vi "All_stats.vi"(3 "Timescales":dbl[](array[numeric]), 4 "Equi Spaced":dbl[][](array[numeric]) format="%.2f", 5 "LDA":dbl[][](array[numeric]) format="%.2f") -> (1 "Stats array":string[](array[string]))   [LabVIEW 2010]
uses:
  Globals/LDA_meas_global_1.vi
  Globals/Meas_global.vi
  Acquisition/PWA/PWAtasksGLOBAL.vi
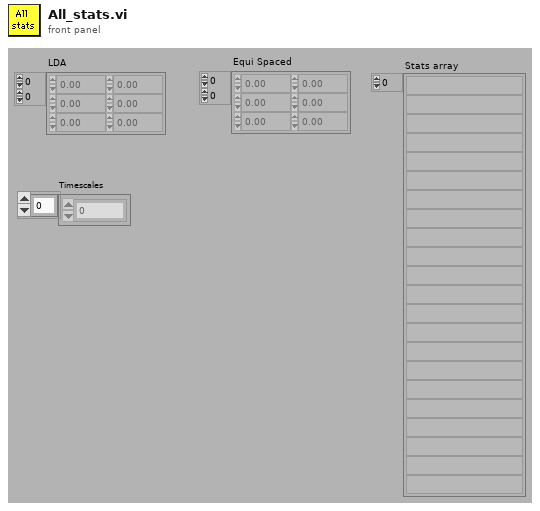
[diagram p1: front panel]
types:
  T1 = typedef "Analysis_type_cluster.ctl" = cluster{"Analysis type":T2, "Indicies":i32[], "Name":string, "Inst Array":T3, "Info index":i32}
  T2 = typedef "Analysis_type_Enum.ctl" = enum16{"Slow Response", "Fast Response", "Weighted Fast Response", "Fast FID", "Weighted Fast FID", "Cross Wire", "Weighted Cross Wire", "Weighted LDA"}
  T3 = typedef "Instrument_Array.ctl" = enum16{"PWA", "LDA", "Analogue"}
  T4 = typedef "Analysis_info_cluster.ctl" = cluster{"Colour":u32, "Inst type":T5, "Inst name":string, "Symbol":string, "Code name":string, "Extra Info":string, "Inst Array":T3, "Index":i32, "Voltage Index":i32, "Extra Titles":string[], "Extra Values":string[]}
  T5 = typedef "Inst_type.ctl" = enum16{"Propeller anemometer", "Raw voltage", "Pressure Transducer", "Pitot-static tube", "Preston tube", "Hot wire", "Cross wire 1", "Cross wire 2", "Generic Linear", "Generic Polynomial", "Generic BackPoly", "Fast FID", "Thermocouple", "Cold wire", "Pulsed Wire", "LDA Vel", "LDA Tran time", "LDA Arr time"}
  T6 = typedef "Velocity_cluster.ctl" = cluster{"Name":string, "U":dbl, "u^2":dbl, "u^3/(u^2)^(1.5)":dbl, "u^4/(u^2)^2 -3":dbl, "% u'/U":dbl, "Mean % Err":dbl, "u^4":dbl}
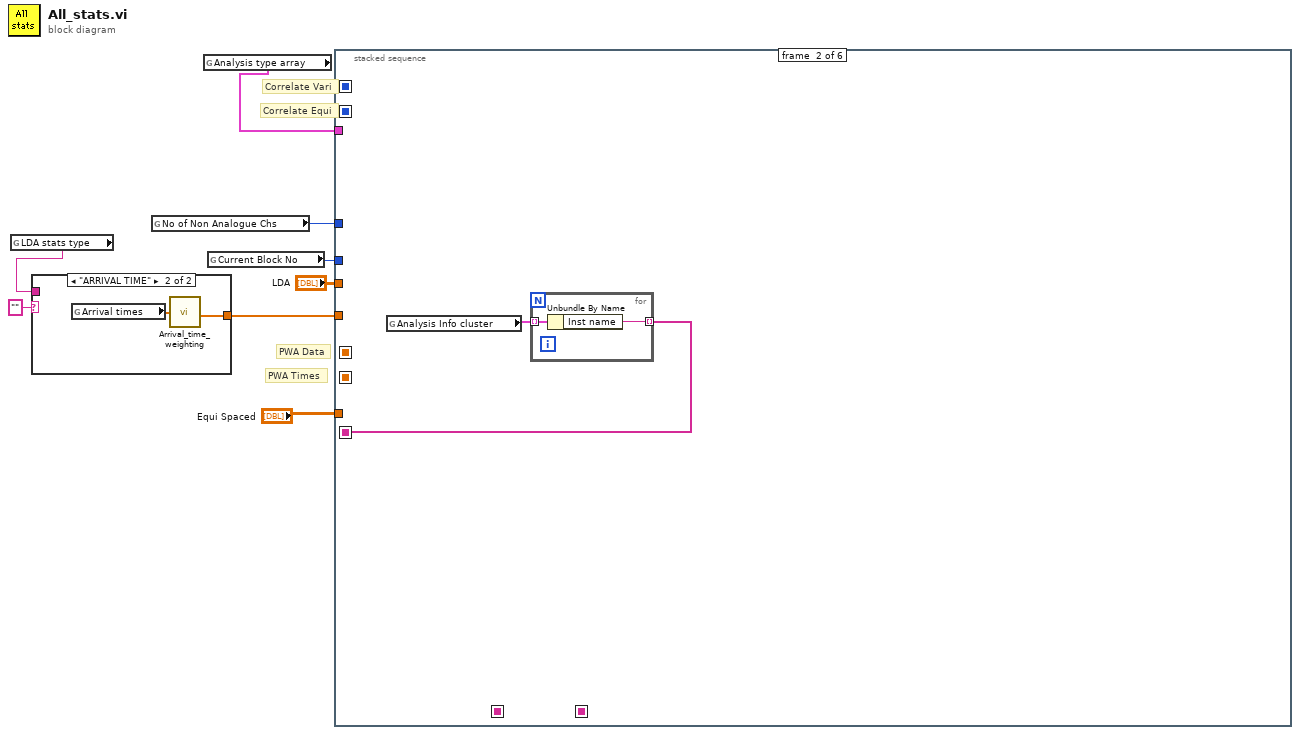
[diagram p0: block diagram]
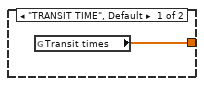
[diagram p2: hidden frame]
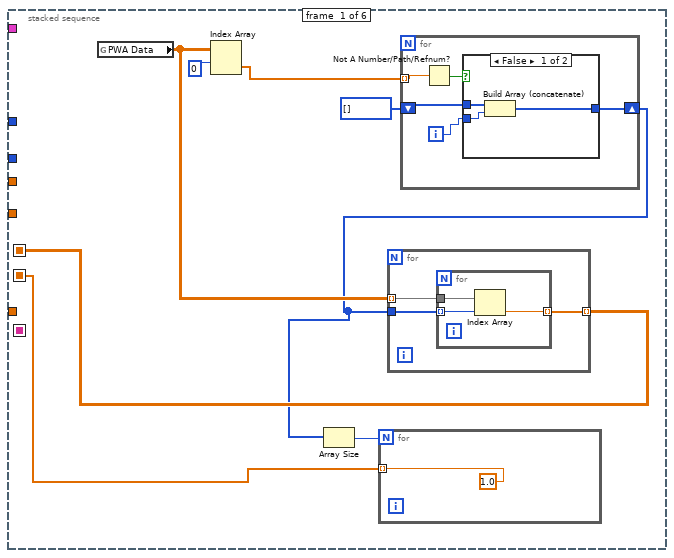
[diagram p3: hidden frame]
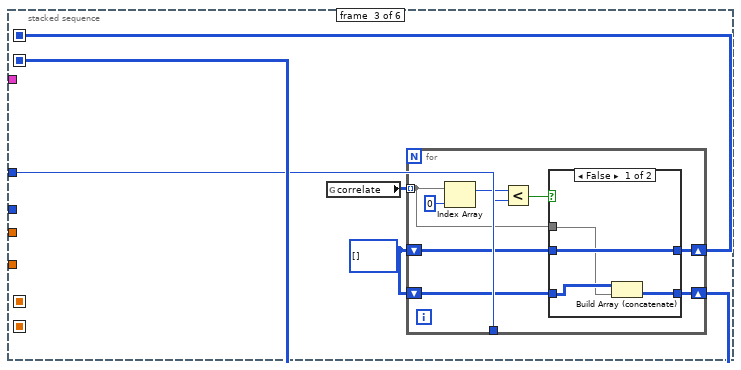
[diagram p5: hidden frame]
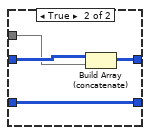
[diagram p6: hidden frame]
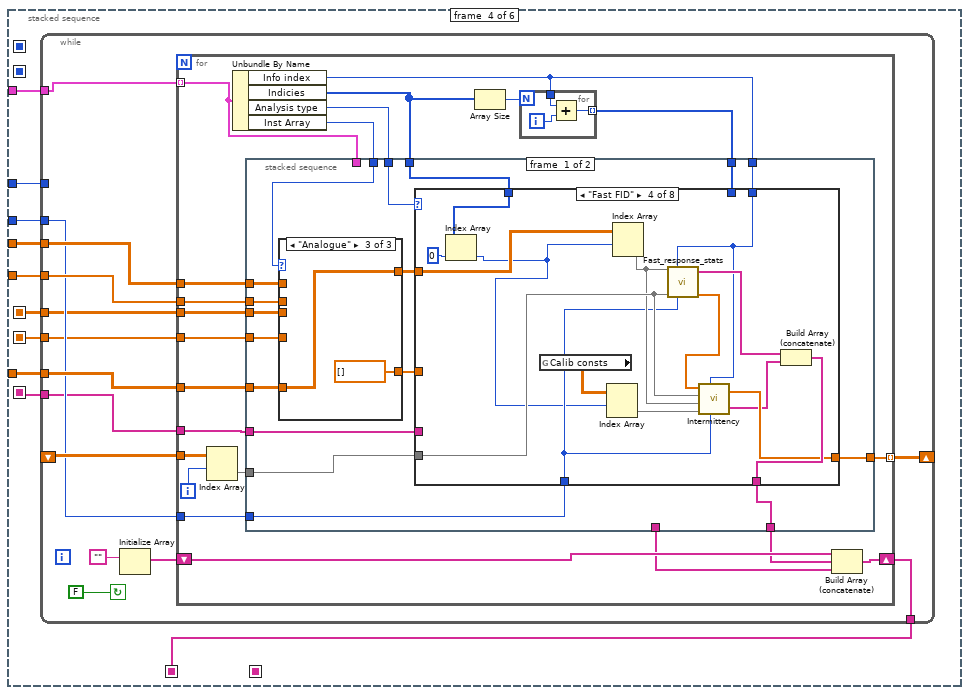
[diagram p7: hidden frame]
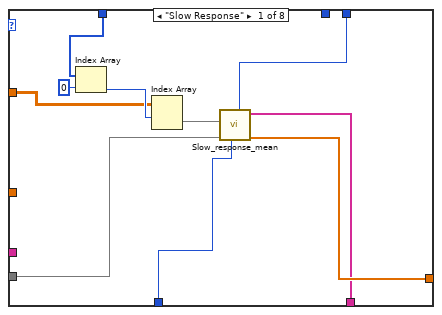
[diagram p10: hidden frame]
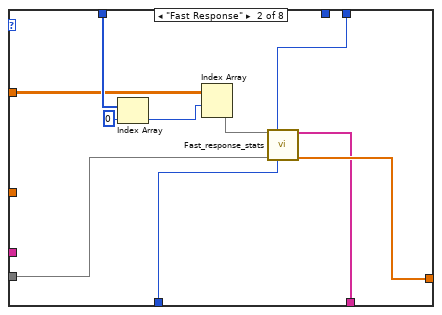
[diagram p11: hidden frame]
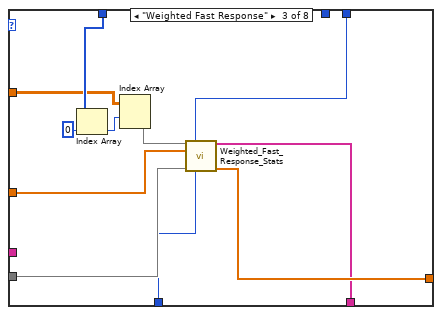
[diagram p12: hidden frame]
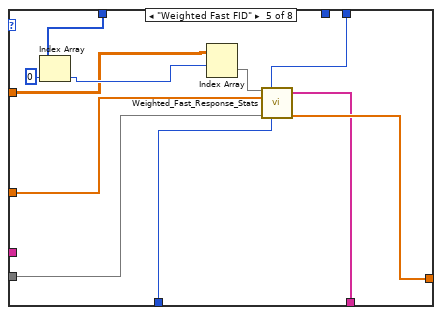
[diagram p13: hidden frame]
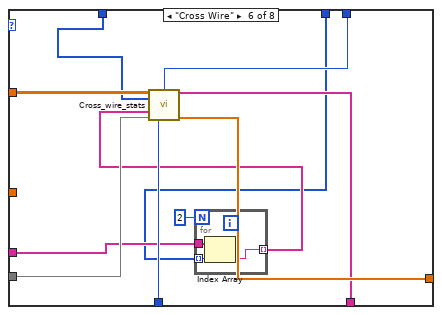
[diagram p14: hidden frame]
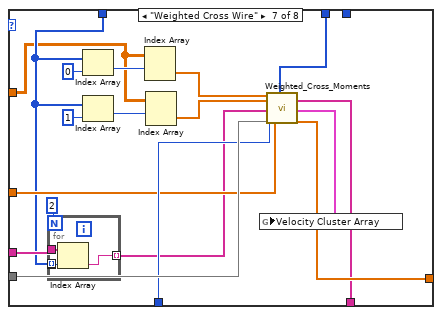
[diagram p15: hidden frame]
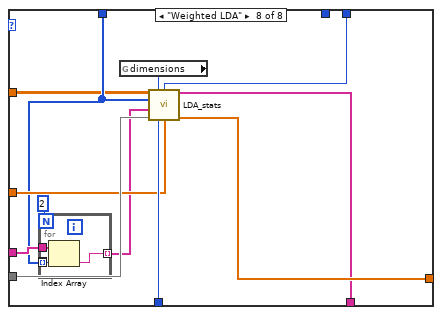
[diagram p16: hidden frame]
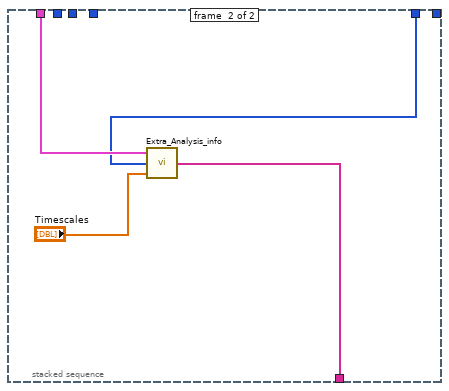
[diagram p17: hidden frame]
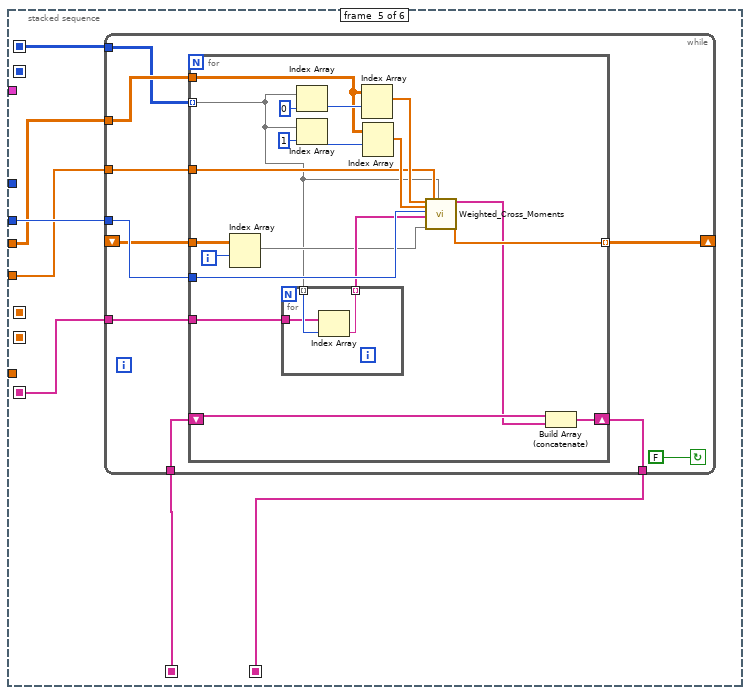
[diagram p18: hidden frame]
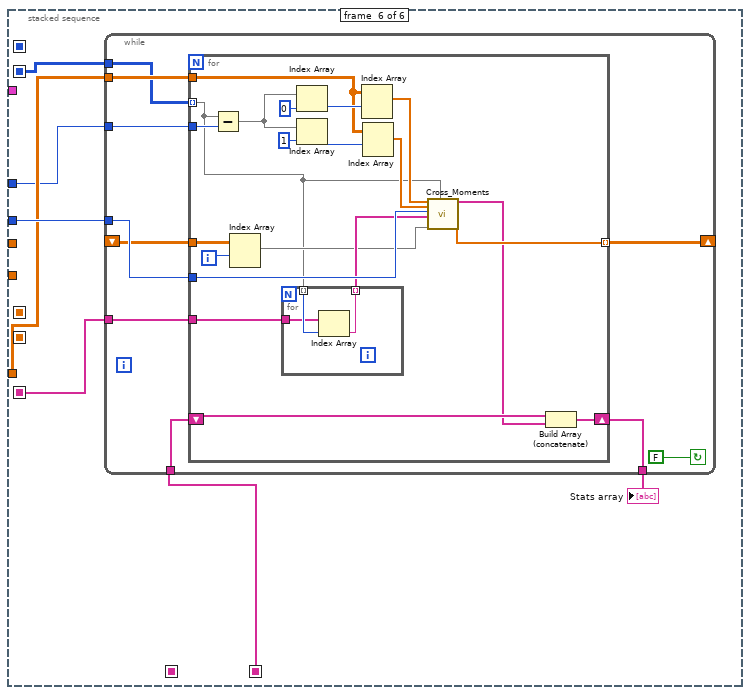
[diagram p19: hidden frame]
diagram:
  # "PWA Times"
  # "PWA Data"
  # "Correlate Equi"
  # "Correlate Vari"
  n1 = global read "LDA_meas_global_1.vi" "LDA stats type"() -> (w1:string)
  n2 = case shown="\"ARRIVAL TIME\"" "" {
    tunnel: [w9 w10] -> w4
    tunnel: w1 -> [_ _]
    frame "TRANSIT TIME", Default {
      n3 = global read "LDA_meas_global_1.vi" "Transit times"() -> (w9:dbl[])
    }
    frame "ARRIVAL TIME" {
      n4 = global read "LDA_meas_global_1.vi" "Arrival times"() -> (w11:dbl[])
      n5 = call "Arrival_time_weighting.vi"("Arrival times"=w11) -> ("Weighting"=w10:dbl[])
    }
  }
  n6 = global read "Meas_global.vi" "No of Non Analogue Chs"() -> (w5:i32)
  n7 = global read "Meas_global.vi" "Analysis type array"() -> (w3:T1[])
  n8 = global read "Meas_global.vi" "Current Block No"() -> (w8:i32)
  n9 = stacked-sequence {
    seq-local: [_ _ _ w69 _ _] -> [_ _ _ _ w249 _]
    seq-local: [_ w36 _ _ _ _] -> [_ _ _ w66 w246 w289]
    seq-local: [_ _ w42 _ _ _] -> [_ _ _ _ w248 _]
    seq-local: [_ _ w41 _ _ _] -> [_ _ _ _ _ w286]
    seq-local: [_ _ _ _ w247 _] -> [_ _ _ _ _ w288]
    seq-local: [w15 _ _ _ _ _] -> [_ _ _ w63 _ _]
    seq-local: [w12 _ _ _ _ _] -> [_ _ _ w62 _ _]
    tunnel: w8 -> [_ _ _ w71 w251 w290]
    tunnel: "LDA" -> [_ _ _ w70 w250 _]
    tunnel: "Equi Spaced" -> [_ _ _ w68 _ w285]
    tunnel: w4 -> [_ _ _ w67 w245 _]
    tunnel: w5 -> [_ _ w40 w64 _ w284]
    tunnel: w3 -> [_ _ _ w65 _ _]
    frame #0 {
      n10 = global read "PWAtasksGLOBAL.vi" "PWA Data"() -> (w16:dbl[][])
      n11 = Index Array(array=w16, index (row)=0) -> (element=w18:dbl[])  [unwired: 1 in]
      n12 = for {
        tunnel: w18 -> [w28] mode=indexing
        shift-right: [w30] -> w14
        shift-left: i32[] [] -> [w31]
        i -> [w27]
        n13 = Not A Number/Path/Refnum?(number/path/refnum=w28) -> (NaN/Path/Refnum?=w29:bool)
        n14 = case shown="False" w29 {
          tunnel: w31 -> [w34 w35]
          tunnel: [w33 w35] -> w30
          tunnel: w27 -> [w32 _]
          frame False {
            n15 = Build Array (concatenate)(w34, w32) -> (w33:i32[])
          }
          frame True {
          }
        }
      }
      n16 = Array Size(array=w14) -> (size(s)=w13:i32)
      n17 = for {
        N: w13 -> [_]
        tunnel: [1.0] -> w12 mode=indexing
      }
      n18 = for {
        tunnel: w14 -> [w23]
        tunnel: w16 -> [w22] mode=indexing
        tunnel: [w21] -> w15 mode=indexing
        n19 = for {
          tunnel: w23 -> [w26] mode=indexing
          tunnel: w22 -> [w25]
          tunnel: [w24] -> w21 mode=indexing
          n20 = Index Array(array=w25, index=w26) -> (element=w24:dbl)
        }
      }
    }
    frame #1 {
      n21 = global read "Meas_global.vi" "Analysis Info cluster"() -> (w37:T4[])
      n22 = for {
        tunnel: w37 -> [w39] mode=indexing
        tunnel: [w38] -> w36 mode=indexing
        n23 = Unbundle By Name(w39) -> ("Inst name"=w38:string)
      }
    }
    frame #2 {
      w43 = i32[][] []
      n24 = global read "Meas_global.vi" "correlate"() -> (w44:i32[][])
      n25 = for {
        tunnel: w44 -> [w49] mode=indexing
        tunnel: w40 -> [w45]
        shift-right: [w48] -> w42
        shift-left: w43 -> [w50]
        shift-right: [w46] -> w41
        shift-left: w43 -> [w47]
        n26 = Index Array(array=w49, index=0 ("Index")) -> (element=w52:i32)
        n27 = Less?(x=w52, y=w45) -> (x < y?=w51:bool)
        n28 = case shown="False" w51 {
          tunnel: w50 -> [w55 w61]
          tunnel: w49 -> [w54 w60]
          tunnel: [w55 w59] -> w48
          tunnel: w47 -> [w57 w58]
          tunnel: [w56 w58] -> w46
          frame False {
            n29 = Build Array (concatenate)(w57, w54) -> (w56:i32[][])
          }
          frame True {
            n30 = Build Array (concatenate)(w61, w60) -> (w59:i32[][])
          }
        }
      }
    }
    frame #3 {
      n31 = while {
        tunnel: w66 -> [w76]
        tunnel: w67 -> [w79]
        tunnel: w68 -> [w81]
        tunnel: [w82] -> w69
        shift-left: _ -> [w78]
        shift-right: [w85] -> _
        tunnel: w70 -> [w80]
        tunnel: w71 -> [w77]
        tunnel: w65 -> [w74]
        tunnel: w64 -> [_]
        tunnel: w63 -> [w73]
        tunnel: w62 -> [w72]
        stop <- FALSE continue-if-true
        n32 = Initialize Array("") -> (w83:string[])  [unwired: 1 out]
        n33 = for {
          tunnel: w80 -> [w92]
          tunnel: [w106] -> w85 mode=indexing
          tunnel: w77 -> [w105]
          shift-right: [w104] -> w82
          shift-left: w83 -> [w103]
          tunnel: w81 -> [w101]
          tunnel: w79 -> [w100]
          tunnel: w78 -> [w99]
          tunnel: w76 -> [w96]
          tunnel: w74 -> [w95] mode=indexing
          tunnel: w73 -> [w91]
          tunnel: w72 -> [w90]
          i -> [w97]
          n34 = Index Array(array=w99, index (row)=w97) -> (element=w98:dbl[])  [unwired: 1 in]
          n35 = Unbundle By Name(w95) -> ("Info index"=w88:i32, "Indicies"=w89:i32[], "Analysis type"=w107:T2, "Inst Array"=w93:T3)
          n36 = Array Size(array=w89) -> (size(s)=w87:i32)
          n37 = for {
            N: w87 -> [_]
            tunnel: w88 -> [w109]
            tunnel: [w108] -> w86 mode=indexing
            i -> [w110]
            n38 = Add(x=w109, y=w110) -> (x+y=w108:i32)
          }
          n39 = stacked-sequence {
            tunnel: w107 -> [w127 _]
            tunnel: w89 -> [w126 _]
            tunnel: [w125 _] -> w106
            tunnel: w105 -> [w124 _]
            tunnel: [w123 _] -> w102
            tunnel: w101 -> [w115 _]
            tunnel: w100 -> [w116 _]
            tunnel: w98 -> [w122 _]
            tunnel: w96 -> [w121 _]
            tunnel: w95 -> [_ w244]
            tunnel: [_ w242] -> w94
            tunnel: w93 -> [w120 _]
            tunnel: w92 -> [w119 _]
            tunnel: w91 -> [w114 _]
            tunnel: w90 -> [w113 _]
            tunnel: w88 -> [w112 _]
            tunnel: w86 -> [w111 w241]
            frame #0 {
              n40 = case shown="\"Analogue\"" w120 {
                tunnel: w119 -> [_ w131 _]
                tunnel: [w129 w131 w133] -> w118
                tunnel: [w128 w130 dbl[] [] ("Weighting")] -> w117
                tunnel: w116 -> [_ w130 _]
                tunnel: w115 -> [_ _ w133]
                tunnel: w114 -> [w129 _ _]
                tunnel: w113 -> [w128 _ _]
                frame "PWA" {
                }
                frame "LDA" {
                }
                frame "Analogue" {
                }
              }
              n41 = case shown="\"Fast FID\"" w127 {
                tunnel: w126 -> [w138 w152 w163 w178 w189 w193 w211 w229]
                tunnel: w122 -> [w140 w147 w160 w173 w186 w200 w221 w236]
                tunnel: [w141 w150 w161 w170 w187 w201 w222 w237] -> w125
                tunnel: w124 -> [w139 w149 w159 w168 w185 w199 w220 w235]
                tunnel: [w137 w148 w157 w175 w182 w198 w205 w234] -> w123
                tunnel: w117 -> [_ _ w156 _ w184 _ w219 w232]
                tunnel: w121 -> [_ _ _ _ _ w196 w216 w230]
                tunnel: w118 -> [w135 w146 w155 w167 w181 w194 w210 w227]
                tunnel: w112 -> [w134 w145 w154 w165 w180 w192 _ w226]
                tunnel: w111 -> [_ _ _ _ _ w191 w206 _]
                frame "Slow Response" {
                  n42 = Index Array(array=w138, index=0) -> (element=w136:i32)
                  n43 = Index Array(array=w135, index (row)=w136) -> (element=w142:dbl[])  [unwired: 1 in]
                  n44 = call "Slow_response_mean.vi"("Index"=w134, "Block No"=w139, "Shift in"=w140, "U"=w142) -> ("Shift out"=w141:dbl[], "Results file string array"=w137:string[])  [unwired: 4 out]
                }
                frame "Fast Response" {
                  n45 = Index Array(array=w152, index=0) -> (element=w144:i32)
                  n46 = Index Array(array=w146, index (row)=w144) -> (element=w151:dbl[])  [unwired: 1 in]
                  n47 = call "Fast_response_stats.vi"("U"=w151, "Index"=w145, "Shift in"=w147, "Block No"=w149) -> ("Results file string array"=w148:string[], "Shift out"=w150:dbl[])  [unwired: 10 out]
                }
                frame "Weighted Fast Response" {
                  n48 = Index Array(array=w163, index=0) -> (element=w158:i32)
                  n49 = Index Array(array=w155, index (row)=w158) -> (element=w162:dbl[])  [unwired: 1 in]
                  n50 = call "Weighted_Fast_Response_Stats.vi"("U"=w162, "Index"=w154, "Weighting"=w156, "Shift in"=w160, "Block No"=w159) -> ("Results file string array"=w157:string[], "Shift out"=w161:dbl[])  [unwired: 1 in, 8 out]
                }
                frame "Fast FID" {
                  n51 = Index Array(array=w178, index=0) -> (element=w166:i32)
                  n52 = global read "Meas_global.vi" "Calib consts"() -> (w177:dbl[][])
                  n53 = Index Array(array=w177, index (row)=w166) -> (element=w171:dbl[])  [unwired: 1 in]
                  n54 = Index Array(array=w167, index (row)=w166) -> (element=w172:dbl[])  [unwired: 1 in]
                  n55 = call "Fast_response_stats.vi"("U"=w172, "Index"=w165, "Shift in"=w173, "Block No"=w168) -> ("Results file string array"=w176:string[], "Shift out"=w174:dbl[])  [unwired: 10 out]
                  n56 = call "Intermittency.vi"("Block No"=w168, "Index"=w165, "Calib Constants"=w171, "C"=w172, "Shift in Before Fast Response"=w173, "Shift in After Fast Response"=w174) -> ("Results"=w169:string[], "Shift Out"=w170:dbl[])
                  n57 = Build Array (concatenate)(w176, w169) -> (w175:string[])
                }
                frame "Weighted Fast FID" {
                  n58 = Index Array(array=w189, index=0) -> (element=w183:i32)
                  n59 = Index Array(array=w181, index (row)=w183) -> (element=w188:dbl[])  [unwired: 1 in]
                  n60 = call "Weighted_Fast_Response_Stats.vi"("U"=w188, "Index"=w180, "Weighting"=w184, "Shift in"=w186, "Block No"=w185) -> ("Results file string array"=w182:string[], "Shift out"=w187:dbl[])  [unwired: 1 in, 8 out]
                }
                frame "Cross Wire" {
                  n61 = for {
                    N: 2 -> [_]
                    tunnel: w196 -> [w204]
                    tunnel: w191 -> [w203] mode=indexing
                    tunnel: [w202] -> w195 mode=indexing
                    n62 = Index Array(array=w204, index=w203) -> (element=w202:string)
                  }
                  n63 = call "Cross_wire_stats.vi"("Eng Units"=w194, "Info Index"=w192, "Indicies"=w193, "Inst names"=w195, "Shift in"=w200, "Block No"=w199) -> ("Results file string array"=w198:string[], "Shift out"=w201:dbl[])  [unwired: 2 in, 6 out]
                }
                frame "Weighted Cross Wire" {
                  n64 = for {
                    N: 2 -> [_]
                    tunnel: w216 -> [w225]
                    tunnel: [w223] -> _ mode=indexing
                    tunnel: [w224] -> w217 mode=indexing
                    tunnel: w211 -> [w223] mode=indexing
                    n65 = Index Array(array=w225, index=w223) -> (element=w224:string)
                  }
                  n66 = Index Array(array=w211, index=0) -> (element=w213:i32)
                  n67 = Index Array(array=w211, index=1) -> (element=w212:i32)
                  n68 = Index Array(array=w210, index (row)=w213) -> (element=w208:dbl[])  [unwired: 1 in]
                  n69 = Index Array(array=w210, index (row)=w212) -> (element=w209:dbl[])  [unwired: 1 in]
                  n70 = call "Weighted_Cross_Moments.vi"("U"=w208, "W"=w209, "Block No"=w220, "Inst names"=w217, "Shift in"=w221, "Weighting"=w219, "Indicies"=w206) -> ("All Results for file"=w205:string[], "Velocity Cluster Array Out"=w207:T6[], "Shift out"=w222:dbl[])  [unwired: 1 in, 9 out]
                  n71 = global write "Meas_global.vi" "Velocity Cluster Array"(w207) -> ()
                }
                frame "Weighted LDA" {
                  n72 = for {
                    N: 2 -> [_]
                    tunnel: w230 -> [w240]
                    tunnel: [w239] -> w228 mode=indexing
                    tunnel: [w238] -> _ mode=indexing
                    tunnel: w229 -> [w238] mode=indexing
                    n73 = Index Array(array=w240, index=w238) -> (element=w239:string)
                  }
                  n74 = global read "Meas_global.vi" "dimensions"() -> (w233:enum16{"1D", "2D"})
                  n75 = call "LDA_stats.vi"("Eng Units"=w227, "dimensions"=w233, "Info Index"=w226, "Indicies"=w229, "Inst names"=w228, "Shift in"=w236, "Block No"=w235, "Weighting"=w232) -> ("Results file string array"=w234:string[], "Shift out"=w237:dbl[])  [unwired: 1 in, 5 out]
                }
              }
            }
            frame #1 {
              n76 = call "Extra_Analysis_info.vi"("Timescales"="Timescales", "Indicies"=w241, "Analysis type cluster"=w244) -> ("Values"=w242:string[])
            }
          }
          n77 = Build Array (concatenate)(w103, w102, w94) -> (w104:string[])
        }
      }
    }
    frame #4 {
      n78 = while {
        tunnel: w245 -> [w253]
        tunnel: w246 -> [w254]
        tunnel: w249 -> [w257]
        tunnel: w248 -> [w259]
        tunnel: [w260] -> w247
        shift-left: _ -> [w255]
        shift-right: [w258] -> _
        tunnel: w250 -> [w261]
        tunnel: w251 -> [w256]
        stop <- FALSE continue-if-true
        n79 = for {
          tunnel: w261 -> [w274]
          tunnel: w256 -> [w271]
          shift-right: [w280] -> w260
          shift-left: w257 -> [w279]
          tunnel: w259 -> [w262] mode=indexing
          tunnel: [w270] -> w258 mode=indexing
          tunnel: w254 -> [w268]
          tunnel: w255 -> [w265]
          tunnel: w253 -> [w263]
          i -> [w266]
          n80 = Index Array(array=w265, index (row)=w266) -> (element=w264:dbl[])  [unwired: 1 in]
          n81 = for {
            tunnel: w262 -> [w283] mode=indexing
            tunnel: w268 -> [w282]
            tunnel: [w281] -> w267 mode=indexing
            n82 = Index Array(array=w282, index=w283) -> (element=w281:string)
          }
          n83 = Index Array(array=w262, index=0) -> (element=w276:i32)
          n84 = Index Array(array=w262, index=1) -> (element=w275:i32)
          n85 = Index Array(array=w274, index (row)=w276) -> (element=w273:dbl[])  [unwired: 1 in]
          n86 = Index Array(array=w274, index (row)=w275) -> (element=w272:dbl[])  [unwired: 1 in]
          n87 = call "Weighted_Cross_Moments.vi"("U"=w273, "W"=w272, "Block No"=w271, "Inst names"=w267, "Shift in"=w264, "Weighting"=w263, "Indicies"=w262) -> ("Correlations Only"=w269:string[], "Shift out"=w270:dbl[])  [unwired: 1 in, 10 out]
          n88 = Build Array (concatenate)(w279, w269) -> (w280:string[])
        }
      }
    }
    frame #5 {
      n89 = while {
        tunnel: w284 -> [w292]
        tunnel: w289 -> [w293]
        tunnel: w288 -> [w296]
        tunnel: w286 -> [w298]
        tunnel: [w299] -> w287
        shift-left: _ -> [w294]
        shift-right: [w297] -> _
        tunnel: w285 -> [w300]
        tunnel: w290 -> [w295]
        stop <- FALSE continue-if-true
        n90 = for {
          tunnel: w300 -> [w314]
          tunnel: w295 -> [w311]
          shift-right: [w320] -> w299
          shift-left: w296 -> [w319]
          tunnel: w298 -> [w301] mode=indexing
          tunnel: [w310] -> w297 mode=indexing
          tunnel: w293 -> [w308]
          tunnel: w294 -> [w305]
          tunnel: w292 -> [w303]
          i -> [w306]
          n91 = Subtract(x=w301, y=w303) -> (x-y=w302:i32[])
          n92 = Index Array(array=w305, index (row)=w306) -> (element=w304:dbl[])  [unwired: 1 in]
          n93 = for {
            tunnel: w301 -> [w323] mode=indexing
            tunnel: w308 -> [w322]
            tunnel: [w321] -> w307 mode=indexing
            n94 = Index Array(array=w322, index=w323) -> (element=w321:string)
          }
          n95 = Index Array(array=w302, index=0) -> (element=w316:i32)
          n96 = Index Array(array=w302, index=1) -> (element=w315:i32)
          n97 = Index Array(array=w314, index (row)=w316) -> (element=w313:dbl[])  [unwired: 1 in]
          n98 = Index Array(array=w314, index (row)=w315) -> (element=w312:dbl[])  [unwired: 1 in]
          n99 = call "Cross_Moments.vi"("U"=w313, "W"=w312, "Block No"=w311, "Inst names"=w307, "Shift in"=w304, "Indicies"=w301) -> ("Correlations Only"=w309:string[], "Shift out"=w310:dbl[])  [unwired: 1 in, 11 out]
          n100 = Build Array (concatenate)(w319, w309) -> (w320:string[])
        }
      }
      "Stats array" <- w287
    }
  }
